vi "Obtain Msg Q.vi"(10 "Alias":string) -> (0 "error out":errorcluster, 3 "Msg Queue out":refnum<class "Msg Q.lvclass">)   [LabVIEW 2021, in "LVCAM.lvlib" / "Msg Q.lvclass"]
uses:
  Msg Q.lvclass
  Msg/Msg.lvclass
  Msg Q.lvclass/Msg Q.ctl
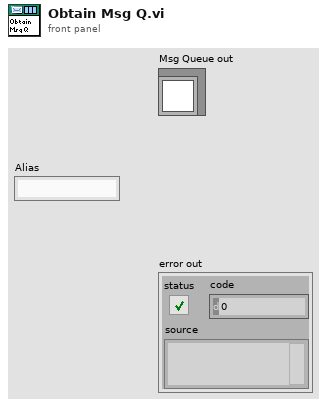
[diagram p1: front panel]
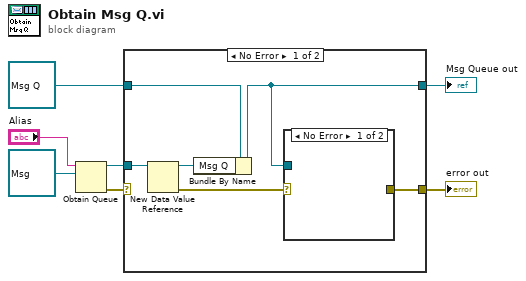
[diagram p0: block diagram]
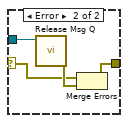
[diagram p2: hidden frame]
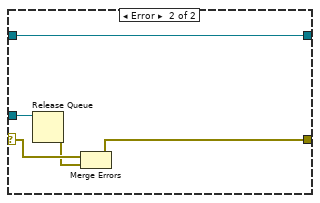
[diagram p3: hidden frame]
diagram:
  n1 = Obtain Queue(name (unnamed)="Alias", element data type=refnum<class "Msg.lvclass"> refnum ("Artifex Actor Model.lvlib:Msg.lvclass")) -> (queue out=w5:refnum<queue>, error out=w6:errorcluster)  [unwired: 3 in, 1 out]
  n2 = case shown="No Error" w6 {
    selector: w6 -> [_ w20]
    tunnel: refnum<class "Msg Q.lvclass"> refnum ("Msg Queue out") -> [w13 w22]
    tunnel: w5 -> [w9 w21]
    tunnel: [w12 w22] -> w2
    tunnel: [w11 w19] -> w1
    frame No Error {
      n3 = New Data Value Reference(data value=w9) -> (data value reference=w8:refnum<data-value>, error out=w10:errorcluster)  [unwired: 1 in]
      n4 = Bundle By Name(cluster=w13, "Msg Q"=w8) -> (w12:refnum<class "Msg Q.lvclass">)
      n5 = case shown="No Error" w10 {
        selector: w10 -> [_ w14]
        tunnel: w12 -> [_ w17]
        tunnel: [_ w16] -> w11
        frame No Error {
        }
        frame Error {
          n6 = call "Release Msg Q.vi"("Msg Queue in"=w17) -> ("error out"=w15:errorcluster)  [unwired: 9 in, 1 out]
          n7 = Merge Errors(w14, w15) -> (w16:errorcluster)
        }
      }
    }
    frame Error {
      n8 = Release Queue(queue=w21) -> (error out=w18:errorcluster)  [unwired: 2 in, 2 out]
      n9 = Merge Errors(w20, w18) -> (w19:errorcluster)
    }
  }
  "Msg Queue out" <- w2
  "error out" <- w1
